vi "MaineReal.vi"   [LabVIEW 2012]
types:
  T1 = cluster{"BoatSpeed":refnum<notifier>, "WindSpeed":refnum<notifier>, "MainPosition":refnum<notifier>, "JibPosition":refnum<notifier>, "MissionCheckOff":refnum<notifier>, "EStop":refnum<notifier>, "SpeedOverWater":refnum<notifier>, "BoatDirection":refnum<notifier>, "RudderPosition":refnum<notifier>, "Luffing":refnum<notifier>, "RudderForce":refnum<notifier>, "BatteryVoltage":refnum<notifier>, "StayForces":refnum<notifier>}
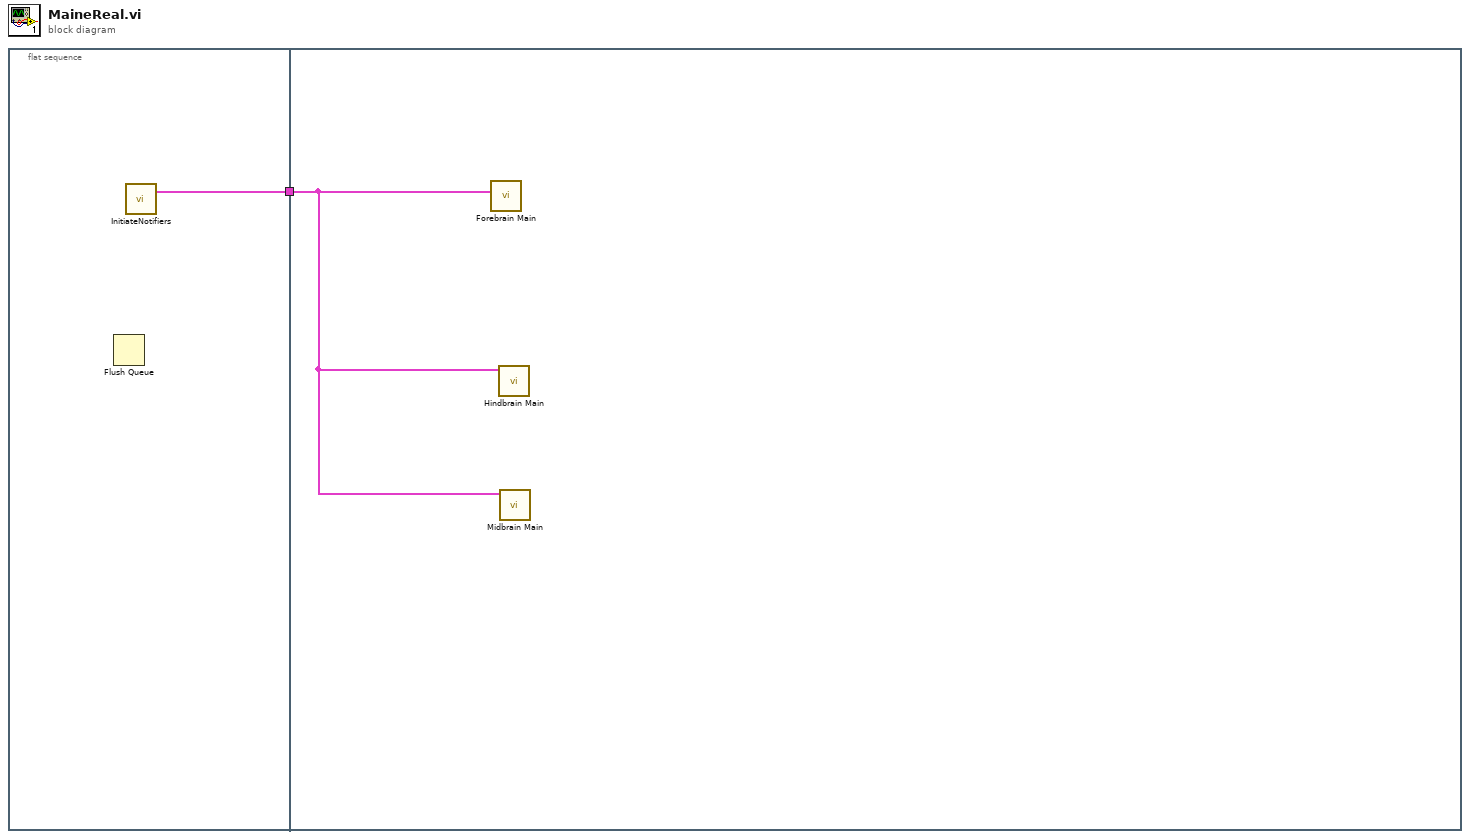
[diagram p0: block diagram]
diagram:
  n1 = flat-sequence {
    tunnel: [w2] -> w1
    tunnel: w1 -> [w3]
    frame #0 {
      n2 = Flush Queue() -> ()  [unwired: 2 in, 3 out]
      n3 = call "InitiateNotifiers.vi"() -> ("NotifierReff"=w2:T1)  [unwired: 2 in, 1 out]
    }
    frame #1 {
      n4 = call "Forebrain Main.vi"("NotifierReff"=w3) -> ()  [unwired: 3 in]
      n5 = call "Hindbrain Main.vi"("NotifierReff"=w3) -> ()  [unwired: 11 in]
      n6 = call "Midbrain Main.vi"("NotifierReff"=w3) -> ()  [unwired: 11 in]
    }
  }
